vi "CPG.vi"(9 "r_slip":dbl=-0.08418393253752732, 10 "Reset":dbl[](array[numeric])=[0.1, 0.8, 0.8], 11 "CPG in":T1={"NoPre"=[0, 3, 2], "Pre IDs"=[0, 1, 2, 1, 2, 2, 4, 1, 3, 4, 2, 3, 4], "W"=[0.0482, 0.77355, 0.5668712995192191, -0.4725094194920492, 0.891141, 0.2729, -0.5705650835351092, -1.0808497974664866, 1.0, -2.220574311751122, -0.9050911281454722, -0.6675323382212381, 0.42449788704559716], "Current"=[0.1, -0.9695973495875724, -0.6516595533946521]}) -> (0 "neuron 2":dbl=-0.6494074649679148, 1 "neuron 1":dbl=-0.9695187557753245, 3 "CPG out":T1={"NoPre"=[0, 3, 2], "Pre IDs"=[0, 1, 2, 1, 2, 2, 4, 1, 3, 4, 2, 3, 4], "W"=[0.0482, 0.77355, 0.5668712995192191, -0.4725094194920492, 0.891141, 0.2729, -0.5705650835351092, -1.0808497974664866, 1.0, -2.220574311751122, -0.9050911281454722, -0.6675323382212381, 0.42449788704559716], "Current"=[0.1, -0.9695187557753245, -0.6494074649679148]})   [LabVIEW 2016]
panel:
  out "M Input":dbl(graph)
  out "W":cluster{"W[0]":dbl, "W[1]":dbl, "W[2]":dbl}(graph)={"W[0]"=0.1, "W[1]"=-0.9695187557753245, "W[2]"=-0.6494074649679148}
  in  "M":dbl[](array[numeric])=[-1e-06, -1e-06]
  in  "x":dbl=1.0
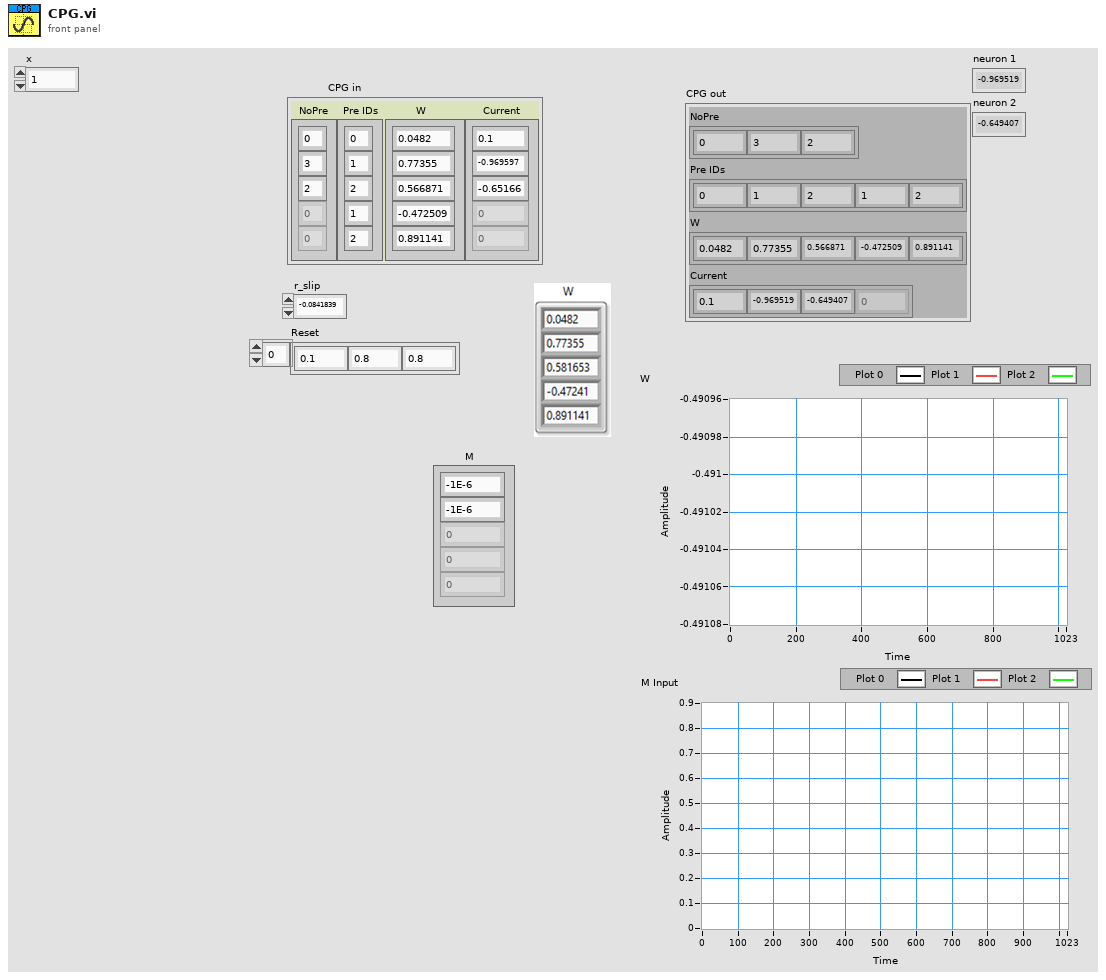
[diagram p1: front panel]
types:
  T1 = cluster{"NoPre":i32[], "Pre IDs":i32[], "W":dbl[], "Current":dbl[]}
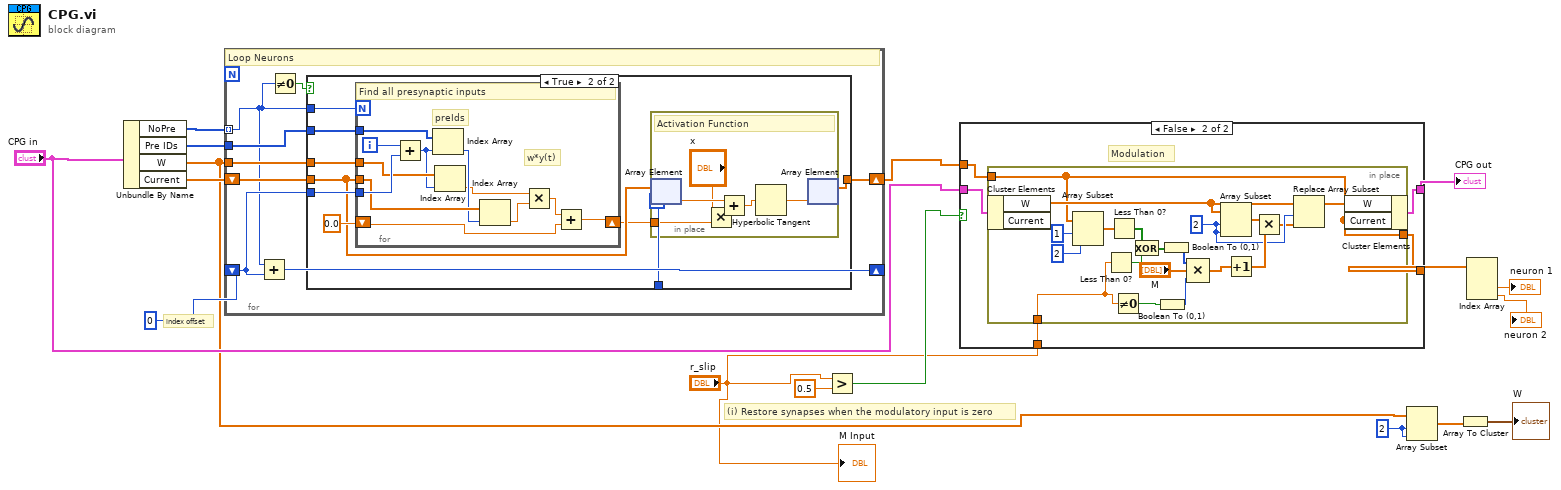
[diagram p0: block diagram]
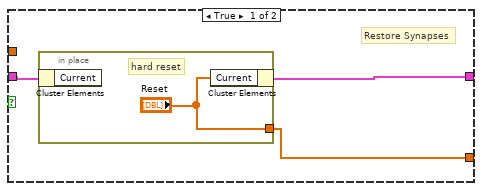
[diagram p2: hidden frame]
diagram:
  w4 = 2 ("index")
  # "(i) Restore synapses when the modulatory input is zero"
  # "index offset"
  n1 = Unbundle By Name("CPG in") -> ("NoPre"=w17:i32[], "Pre IDs"=w15:i32[], "W"=w2:dbl[], "Current"=w14:dbl[])
  n2 = for {
    tunnel: w17 -> [w18] mode=indexing
    shift-right: [w26] -> _
    shift-left: 0 -> [w25]
    tunnel: w15 -> [w24]
    tunnel: w2 -> [w20]
    shift-right: [w21] -> w12
    shift-left: w14 -> [w23]
    i -> [w22]
    # "Loop Neurons"
    n3 = Add(x=w18, y=w25) -> (x+y=w26:i32)
    n4 = Not Equal To 0?(x=w18) -> (x != 0?=w19:bool)
    n5 = case shown="True" w19 {
      tunnel: w18 -> [_ w36]
      tunnel: w25 -> [_ w35]
      tunnel: w24 -> [_ w34]
      tunnel: w23 -> [w27 w32]
      tunnel: w22 -> [_ w31]
      tunnel: [w27 w29] -> w21
      tunnel: w20 -> [_ w28]
      frame False {
      }
      frame True {
        n6 = for {
          N: w36 -> [_]
          tunnel: w35 -> [w53]
          tunnel: w34 -> [w52]
          tunnel: w28 -> [w51]
          tunnel: w32 -> [w50]
          shift-right: [w46] -> w30
          shift-left: 0.0 -> [w44]
          i -> [w54]
          # "w*y(t)"
          # "preIds"
          # "Find all presynaptic inputs"
          n7 = Add(x=w54, y=w53) -> (x+y=w43:i32)
          n8 = Index Array(array=w52, index=w43) -> (element=w49:i32)
          n9 = Index Array(array=w51, index=w43) -> (element=w48:dbl)
          n10 = Index Array(array=w50, index=w49) -> (element=w47:dbl)
          n11 = Multiply(x=w48, y=w47) -> (x*y=w45:dbl)
          n12 = Add(x=w45, y=w44) -> (x+y=w46:dbl)
        }
        n13 = in-place {
          in-place-border: w30 -> [w42]
          # "Activation Function"
          n14 = in-place-array #1(w32, w31) -> (w40:dbl)
          n15 = Multiply(x="x", y=w42) -> (x*y=w38:dbl)
          n16 = Add(x=w40, y=w38) -> (x+y=w39:dbl)
          n17 = Hyperbolic Tangent(1:w39) -> (0:w41:dbl)
          n18 = in-place-array #1(w41) -> (w29:dbl[])  [unwired: 1 out]
        }
      }
    }
  }
  n19 = Greater?(x="r_slip", y=0.5) -> (0:w8:bool)
  n20 = case shown="False" w8 {
    tunnel: "CPG in" -> [w57 w60]
    tunnel: w12 -> [_ w61]
    tunnel: [w56 w63] -> w11
    tunnel: [w55 w62] -> w6
    tunnel: "r_slip" -> [_ w59]
    frame True {
      # "Restore Synapses"
      n21 = in-place {
        in-place-border: ["Reset"] -> w55
        # "hard reset"
        n22 = in-place-cluster #2(w57) -> ()  [unwired: 1 out]
        n23 = in-place-cluster #2("Current"="Reset") -> (w56:T1)
      }
    }
    frame False {
      # "Modulation"
      n24 = in-place {
        in-place-border: w61 -> [w68]
        in-place-border: [w68] -> w62
        in-place-border: w59 -> [w66]
        w76 = 2 ("index")
        n25 = in-place-cluster #3(w60) -> ("W"=w77:dbl[])  [unwired: 1 out]
        n26 = Array Subset(array=w68, index=1, length=2) -> (w71:dbl[])
        n27 = Less Than 0?(x=w66) -> (x < 0?=w70:bool)
        n28 = Less Than 0?(x=w71) -> (x < 0?=w72:bool[])
        n29 = Not Equal To 0?(x=w66) -> (x != 0?=w65:bool)
        n30 = Exclusive Or(1:w70, 2:w72) -> (0:w69:bool[])
        n31 = Boolean To (0,1)(Boolean=w65) -> (0, 1=w64:i16)
        n32 = Boolean To (0,1)(Boolean=w69) -> (0, 1=w82:i16[])
        n33 = Compound Arithmetic op=MULTIPLY(w82, "M", w64) -> (w81:dbl[])
        n34 = Array Subset(array=w77, index=w76, length=w76) -> (w78:dbl[])
        n35 = Increment(x=w81) -> (x+1=w80:dbl[])
        n36 = Multiply(x=w78, y=w80) -> (x*y=w67:dbl[])
        n37 = Replace Array Subset(array=w77, new element=w67, index=w76) -> (w73:dbl[])
        n38 = in-place-cluster #3("W"=w73, "Current"=w68) -> (w63:T1)
      }
    }
  }
  "CPG out" <- w11
  n39 = Array Subset(array=w2, index=w4, length=w4) -> (w3:dbl[])
  n40 = Array To Cluster(array=w3) -> (cluster=→"W":cluster{"[0]":dbl, "[1]":dbl, "[2]":dbl})
  n41 = Index Array(array=w6) -> (element #2=→"neuron 1":dbl, element #3=→"neuron 2":dbl)  [unwired: 3 in, 1 out]
  "M Input" <- "r_slip"
